vi "EvaluateDataFlowBlock.vi"(8 "error in (no error)":errorcluster, 9 "data":T2, 10 "config":T1, 11 "Qbus":refnum<class "Qbus.lvclass">) -> (0 "error out":errorcluster, 2 "config":T1)   [LabVIEW 2017, in "CmsDataEventCreator.lvlib"]
uses:
  <vilib>/addons/InsightCM/Devices/Shared/Cms/CmsDataEventCreator/CmsDataEventCreator.lvlib
  <vilib>/addons/InsightCM/Devices/Shared/Common/DataFlow/controls/Data.ctl
  <vilib>/addons/InsightCM/Utilities/DataAccessors/controls/wfmSGL_DVR.ctl
  <vilib>/addons/PointValueMap/controls/PointMap.ctl
  <vilib>/addons/InsightCM/Devices/Shared/Common/DataFlow/controls/Type.ctl
  <vilib>/addons/InsightCM/Devices/Shared/Cms/CmsDataEventCreator/controls/config.ctl
  <vilib>/addons/Qbus/Qbus.lvclass
  <vilib>/addons/InsightCM/Devices/Shared/Cms/CmsDataEventCreator/controls/DataEventConfig.ctl
  <vilib>/addons/InsightCM/Devices/Shared/Cms/CmsDataEventCreator/controls/AcqParams.ctl
  <vilib>/addons/InsightCM/Devices/Shared/Common/DataAccumulator/controls/AccumulationSettings.ctl
  <vilib>/addons/InsightCM/Devices/Shared/Common/DataAccumulator/controls/accumulationType.ctl
  <vilib>/addons/InsightCM/Devices/Shared/Common/DVRBuffer/controls/BufferLocation.ctl
  <vilib>/addons/InsightCM/Devices/Shared/Common/DataEventCreator/controls/Reason.ctl
  <vilib>/addons/PointValueMap/subVIs/Point_Read_string.vi
  <vilib>/addons/PointValueMap/PointValueMap.lvlib
  <vilib>/addons/InsightCM/Devices/Shared/Common/DataEventCreator/DataEventCreator.lvlib
  <vilib>/addons/InsightCM/Devices/Shared/Common/DVRBuffer/DVRBuffer.lvlib
  <vilib>/addons/InsightCM/Devices/Shared/Common/DataAccumulator/DataAccumulator.lvlib
  <vilib>/addons/InsightCM/Devices/Shared/Common/DataFlow/DataFlow.lvlib
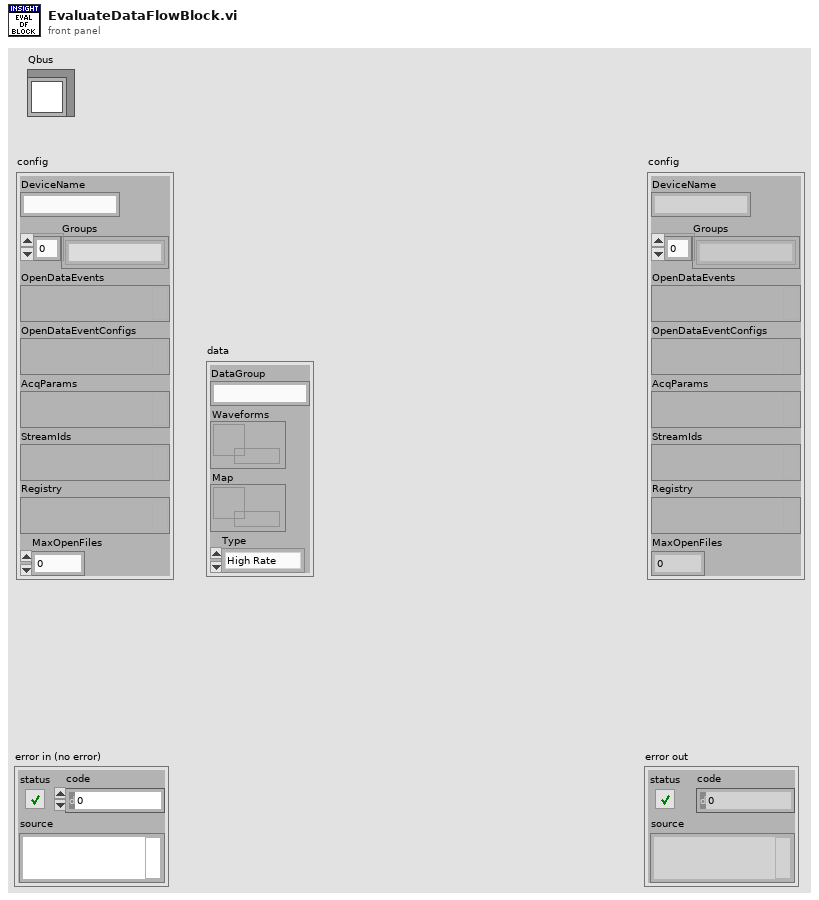
[diagram p1: front panel]
types:
  T1 = typedef "CmsDataEventCreator.lvlib/config.ctl" = cluster{"DeviceName":string, "Groups":string[], "OpenDataEvents":variant, "OpenDataEventConfigs":variant, "AcqParams":variant, "StreamIds":variant, "Registry":variant, "MaxOpenFiles":i32}
  T2 = typedef "DataFlow.lvlib/Data.ctl" = cluster{"DataGroup":string, "Waveforms":T3, "Map":T4, "Type":T5}
  T3 = typedef "wfmSGL_DVR.ctl" = refnum<data-value>
  T4 = typedef "PointValueMap.lvlib/PointMap.ctl" = refnum<data-value>
  T5 = typedef "DataFlow.lvlib/Type.ctl" = enum16{"High Rate", "Low Rate", "Burst Mode"}
  T6 = typedef "CmsDataEventCreator.lvlib/AcqParams.ctl" = cluster{"Stream":bool, "PreTrigger":i32, "CollectOnEnter":bool, "Enter PreTrigger":i32, "Enter Length":dbl, "CollectOnExit":bool, "ContinuousData":bool, "Accumulation Settings":T7}
  T7 = typedef "DataAccumulator.lvlib/AccumulationSettings.ctl" = cluster{"Type":T8, "Length":dbl, "Max Time (sec)":dbl, "Start Block":T9, "Acquired (sec)":dbl, "Acquired (pulses)":i32, "Initial Pulse Offset":dbl, "Stop Block":T9, "LastBlockAdded":u32}
  T8 = typedef "DataAccumulator.lvlib/accumulationType.ctl" = enum16{"none", "seconds", "revolutions"}
  T9 = typedef "DVRBuffer.lvlib/BufferLocation.ctl" = cluster{"Block":u32, "Index":i32}
  T10 = typedef "DataEventCreator.lvlib/Reason.ctl" = enum16{"Periodic Event", "Delta EU Event", "Trend Event", "Alarm Event", "User Event", "Enter Operating State", "Exit Operating State", "Multiple Events", "Other"}
  T11 = typedef "CmsDataEventCreator.lvlib/DataEventConfig.ctl" = cluster{"AcqParams":T6, "OpState":string, "ExitOpState":bool, "Reason":string, "StreamId":string, "Map":T4, "DataSetIds":variant, "IncludeWaveforms":bool, "TrendPointsOnly":bool}
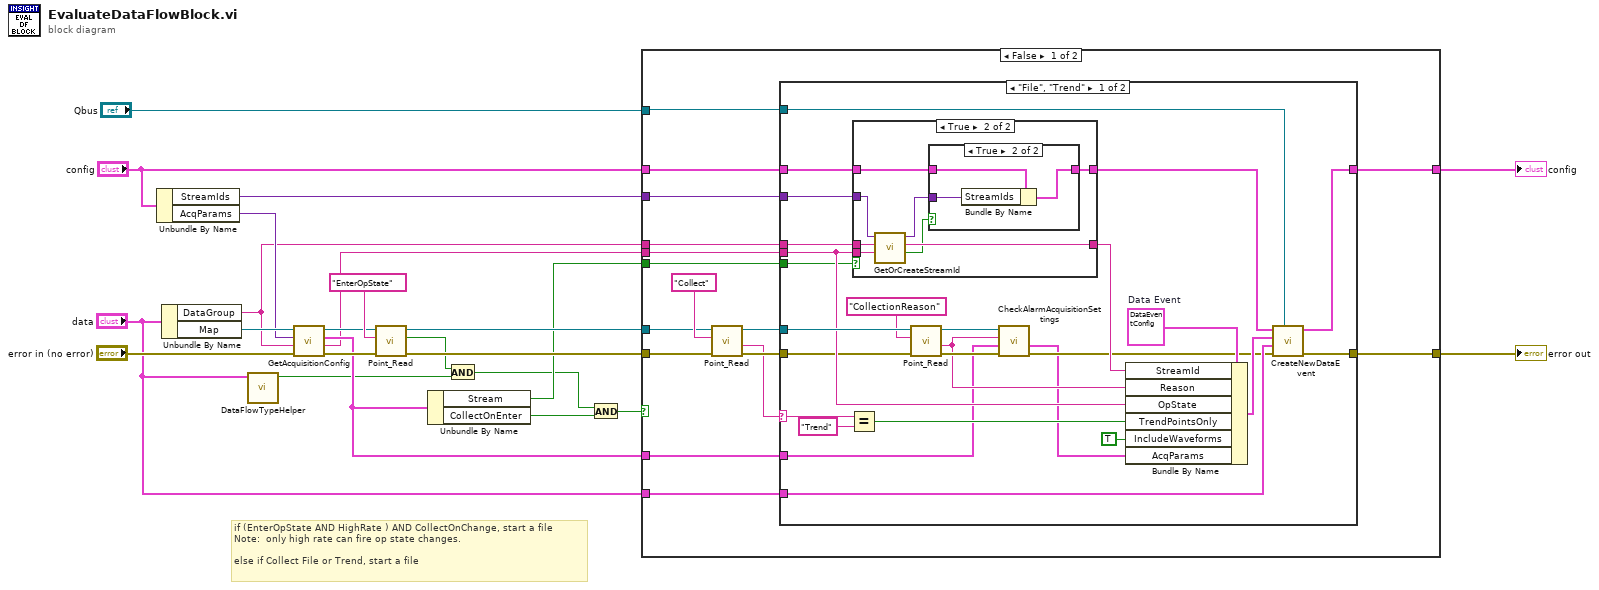
[diagram p0: block diagram]
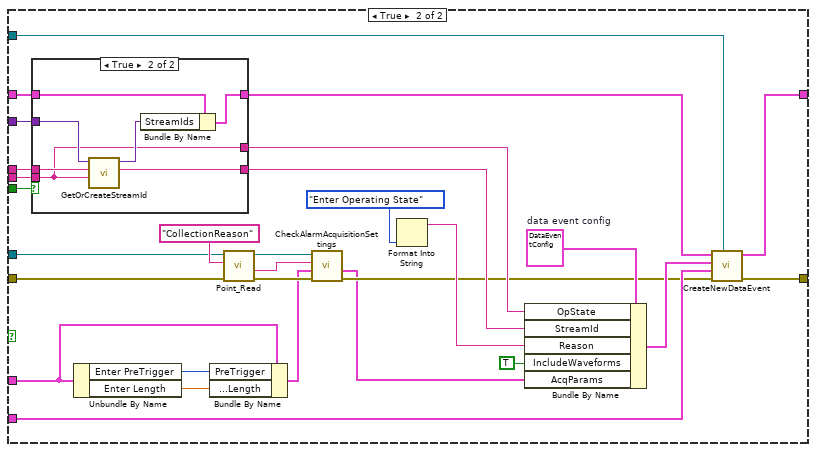
[diagram p5: hidden frame]
diagram:
  # "if (EnterOpState AND HighRate ) AND CollectOnChange, start a file\nNote:  only high rate can fire op state changes.\n\nelse if Collect File or Trend, start a file"
  n1 = Unbundle By Name("config") -> ("StreamIds"=w21:variant, "AcqParams"=w17:variant)
  n2 = Unbundle By Name("data") -> ("DataGroup"=w16:string, "Map"=w18:T4)
  n3 = call <vilib>:"DataFlowTypeHelper.vi"("data"="data") -> ("high rate"=w1:bool)  [unwired: 8 in, 2 out]
  n4 = call <vilib>:"GetAcquisitionConfig.vi"("error in (no error)"="error in (no error)", "DataGroup"=w16, "AcqParams"=w17, "map in"=w18) -> ("error out"=w14:errorcluster, "OpState"=w11:string, "acq config"=w12:T6, "map out"=w13:T4)  [unwired: 4 in]
  n5 = call-poly <vilib>:"Point_Read.vi"("Error In"=w14, "Tag"="EnterOpState", "Map"=w13) -> ("Error Out"=w10:errorcluster, "Found?"=w4:bool, "Map Out"=w8:T4)  [unwired: 3 in, 3 out]
  n6 = Unbundle By Name(w12) -> ("Stream"=w5:bool, "CollectOnEnter"=w7:bool)
  n7 = And(x=w4, y=w1) -> (x .and. y?=w3:bool)
  n8 = And(x=w3, y=w7) -> (x .and. y?=w6:bool)
  n9 = case shown="False" w6 {
    tunnel: [w38 w104] -> w22
    tunnel: w21 -> [w37 w109]
    tunnel: "config" -> [w30 w108]
    tunnel: [w27 w101] -> w19
    tunnel: w16 -> [w26 w107]
    tunnel: w12 -> [w31 w91]
    tunnel: w11 -> [w32 w99]
    tunnel: w10 -> [w35 w86]
    tunnel: "data" -> [w28 w103]
    tunnel: "Qbus" -> [w29 w100]
    tunnel: w8 -> [w36 w85]
    tunnel: w5 -> [w25 w95]
    frame False {
      n10 = call-poly <vilib>:"Point_Read.vi"("Error In"=w35, "Tag"="Collect", "Map"=w36) -> ("Error Out"=w33:errorcluster, "Value"=w24:string, "Map Out"=w34:T4)  [unwired: 3 in, 3 out]
      n11 = case shown="\"File\", \"Trend\"" w24 {
        selector: w24 -> [w48 _]
        tunnel: w34 -> [w65 _]
        tunnel: w33 -> [w55 w80]
        tunnel: [w60 w80] -> w38
        tunnel: w37 -> [w58 _]
        tunnel: w32 -> [w56 _]
        tunnel: w31 -> [w42 _]
        tunnel: w30 -> [w52 w79]
        tunnel: w29 -> [w63 _]
        tunnel: w28 -> [w61 _]
        tunnel: [w59 w79] -> w27
        tunnel: w26 -> [w57 _]
        tunnel: w25 -> [w54 _]
        frame "File", "Trend" {
          w50 = T11 {"AcqParams"={"Stream"=FALSE, "PreTrigger"=0, "CollectOnEnter"=FALSE, "Enter PreTrigger"=0, "Enter Length"=0.0, "CollectOnExit"=FALSE, "ContinuousData"=FALSE, "Accumulation Settings"={"Type"=enum."none", "Length"=0.0, "Max Time (sec)"=0.0, "Start Block"={"Block"=0, "Index"=0}, "Acquired (sec)"=0.0, "Acquired (pulses)"=0, "Initial Pulse Offset"=0.0, "Stop Block"={"Block"=0, "Index"=0}, "LastBlockAdded"=0}}, "OpState"="", "ExitOpState"=FALSE, "Reason"="", "StreamId"="", "Map"=refnum, "DataSetIds"=variant, "IncludeWaveforms"=FALSE, "TrendPointsOnly"=FALSE}  # Data Event
          n12 = Equal?(x=w48, y="Trend") -> (x = y?=w46:bool)
          n13 = case shown="True" w54 {
            tunnel: w58 -> [_ w74]
            tunnel: w57 -> [_ w73]
            tunnel: w56 -> [_ w72]
            tunnel: [_ w71] -> w53
            tunnel: w52 -> [w66 w69]
            tunnel: [w66 w68] -> w51
            frame False {
            }
            frame True {
              n14 = call <vilib>:"GetOrCreateStreamId.vi"("operating state"=w72, "data group"=w73, "stream Ids"=w74) -> ("new streamId"=w67:bool, "stream id"=w71:string, "streamIds out"=w70:variant)  [unwired: 5 in, 1 out]
              n15 = case shown="True" w67 {
                tunnel: w70 -> [_ w78]
                tunnel: w69 -> [w75 w77]
                tunnel: [w75 w76] -> w68
                frame False {
                }
                frame True {
                  n16 = Bundle By Name(cluster=w77, "StreamIds"=w78) -> (w76:T1)
                }
              }
            }
          }
          n17 = call-poly <vilib>:"Point_Read.vi"("Error In"=w55, "Tag"="CollectionReason", "Map"=w65) -> ("Error Out"=w44:errorcluster, "Value"=w43:string, "Map Out"=w41:T4)  [unwired: 3 in, 3 out]
          n18 = call <vilib>:"CheckAlarmAcquisitionSettings.vi"("error in (no error)"=w44, "acq config in"=w42, "collection reason"=w43, "map"=w41) -> ("error out"=w45:errorcluster, "acq config out"=w40:T6)  [unwired: 6 in]
          n19 = Bundle By Name(cluster=w50, "StreamId"=w53, "Reason"=w43, "OpState"=w56, "TrendPointsOnly"=w46, "IncludeWaveforms"=TRUE, "AcqParams"=w40) -> (w62:T11)
          n20 = call <vilib>:"CreateNewDataEvent.vi"("Qbus"=w63, "error in (no error)"=w45, "data flow"=w61, "data event config"=w62, "config"=w51) -> ("error out"=w60:errorcluster, "config out"=w59:T1)  [unwired: 5 in]
        }
        frame Default {
        }
      }
    }
    frame True {
      w96 = T11 {"AcqParams"={"Stream"=FALSE, "PreTrigger"=0, "CollectOnEnter"=FALSE, "Enter PreTrigger"=0, "Enter Length"=0.0, "CollectOnExit"=FALSE, "ContinuousData"=FALSE, "Accumulation Settings"={"Type"=enum."none", "Length"=0.0, "Max Time (sec)"=0.0, "Start Block"={"Block"=0, "Index"=0}, "Acquired (sec)"=0.0, "Acquired (pulses)"=0, "Initial Pulse Offset"=0.0, "Stop Block"={"Block"=0, "Index"=0}, "LastBlockAdded"=0}}, "OpState"="", "ExitOpState"=FALSE, "Reason"="", "StreamId"="", "Map"=refnum, "DataSetIds"=variant, "IncludeWaveforms"=FALSE, "TrendPointsOnly"=FALSE}  # data event config
      n21 = case shown="True" w95 {
        tunnel: w109 -> [_ w118]
        tunnel: w108 -> [w111 w117]
        tunnel: w107 -> [_ w115]
        tunnel: [_ w114] -> w106
        tunnel: w99 -> [w110 w112]
        tunnel: [w111 w113] -> w97
        tunnel: [w110 w112] -> w94
        frame False {
        }
        frame True {
          n22 = call <vilib>:"GetOrCreateStreamId.vi"("operating state"=w112, "data group"=w115, "stream Ids"=w118) -> ("stream id"=w114:string, "streamIds out"=w116:variant)  [unwired: 5 in, 2 out]
          n23 = Bundle By Name(cluster=w117, "StreamIds"=w116) -> (w113:T1)
        }
      }
      n24 = Unbundle By Name(w91) -> ("Enter PreTrigger"=w92:i32, "Enter Length"=w93:dbl)
      n25 = Bundle By Name(cluster=w91, "PreTrigger"=w92, "Accumulation Settings.Length"=w93) -> (w84:T6)
      n26 = call-poly <vilib>:"Point_Read.vi"("Error In"=w86, "Tag"="CollectionReason", "Map"=w85) -> ("Error Out"=w89:errorcluster, "Value"=w88:string, "Map Out"=w87:T4)  [unwired: 3 in, 3 out]
      n27 = call <vilib>:"CheckAlarmAcquisitionSettings.vi"("error in (no error)"=w89, "acq config in"=w84, "collection reason"=w88, "map"=w87) -> ("error out"=w83:errorcluster, "acq config out"=w82:T6)  [unwired: 6 in]
      n28 = Format Into String(Reason."Enter Operating State" ("Reason")) -> (resulting string=w105:string)  [unwired: 3 in, 1 out]
      n29 = Bundle By Name(cluster=w96, "OpState"=w94, "StreamId"=w106, "Reason"=w105, "IncludeWaveforms"=TRUE, "AcqParams"=w82) -> (w102:T11)
      n30 = call <vilib>:"CreateNewDataEvent.vi"("Qbus"=w100, "error in (no error)"=w83, "data flow"=w103, "data event config"=w102, "config"=w97) -> ("error out"=w104:errorcluster, "config out"=w101:T1)  [unwired: 5 in]
    }
  }
  "error out" <- w22
  "config" <- w19
